vi "acquire_dataMultiAxis.vi"(0 "Freq_i":dbl format="%#_13g", 5 "FPGA VI Reference in":refnum<k20>, 7 "error in":errorcluster, 9 "Nsamps_i":i32, 11 "data (sin wave) in":dbl[](array[numeric])) -> (2 "Elements Remaining":i32=1, 4 "FPGA VI Reference Out":refnum<k20>, 6 "error IO":errorcluster, 10 "output cluster":cluster{"z-err data":dbl[], "u_z-data":dbl[]}, 15 "elements left":i32=1)   [LabVIEW 2017]
uses:
  <vilib>/Utility/error.llb/Error Cluster From Error Code.vi
  <vilib>/rvi/errors/niLvFpgaAdjustHostInterfaceError.vi
  <vilib>/rvi/interface/nirviMethod/nirviMethod.xnode
  <vilib>/rvi/errors/niLvFpgaMergeErrorWithErrorCode.vi
  <vilib>/FPGAPlugInAG/Dynamic/niLvFpga_ReadFifo_Dynamic.vi
  <vilib>/FPGAPlugInAG/Dynamic/niLvFpga_WriteFifo_Dynamic.vi
panel:
  out "x+y 2":i32
  out "appended array":i32[](array[numeric])
  out "Numeric 3":i32
  out "Numeric 2":i32
  out "x+y":i32
  out "Numeric":i32
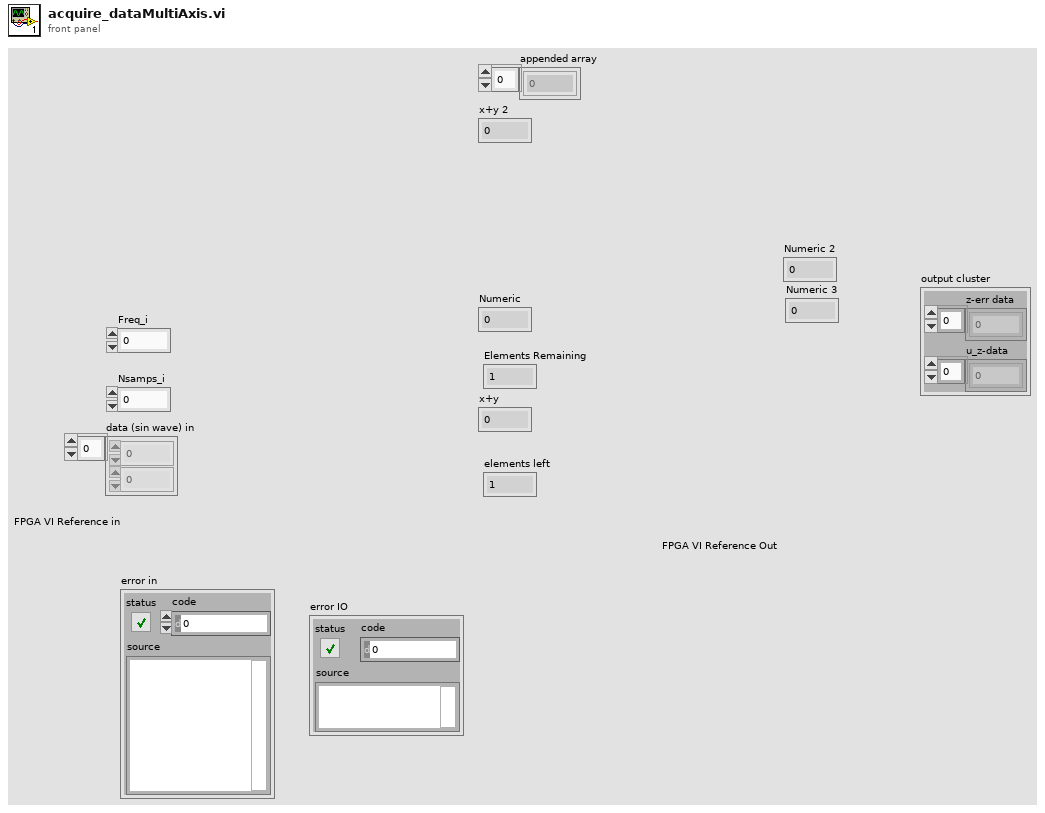
[diagram p1: front panel]
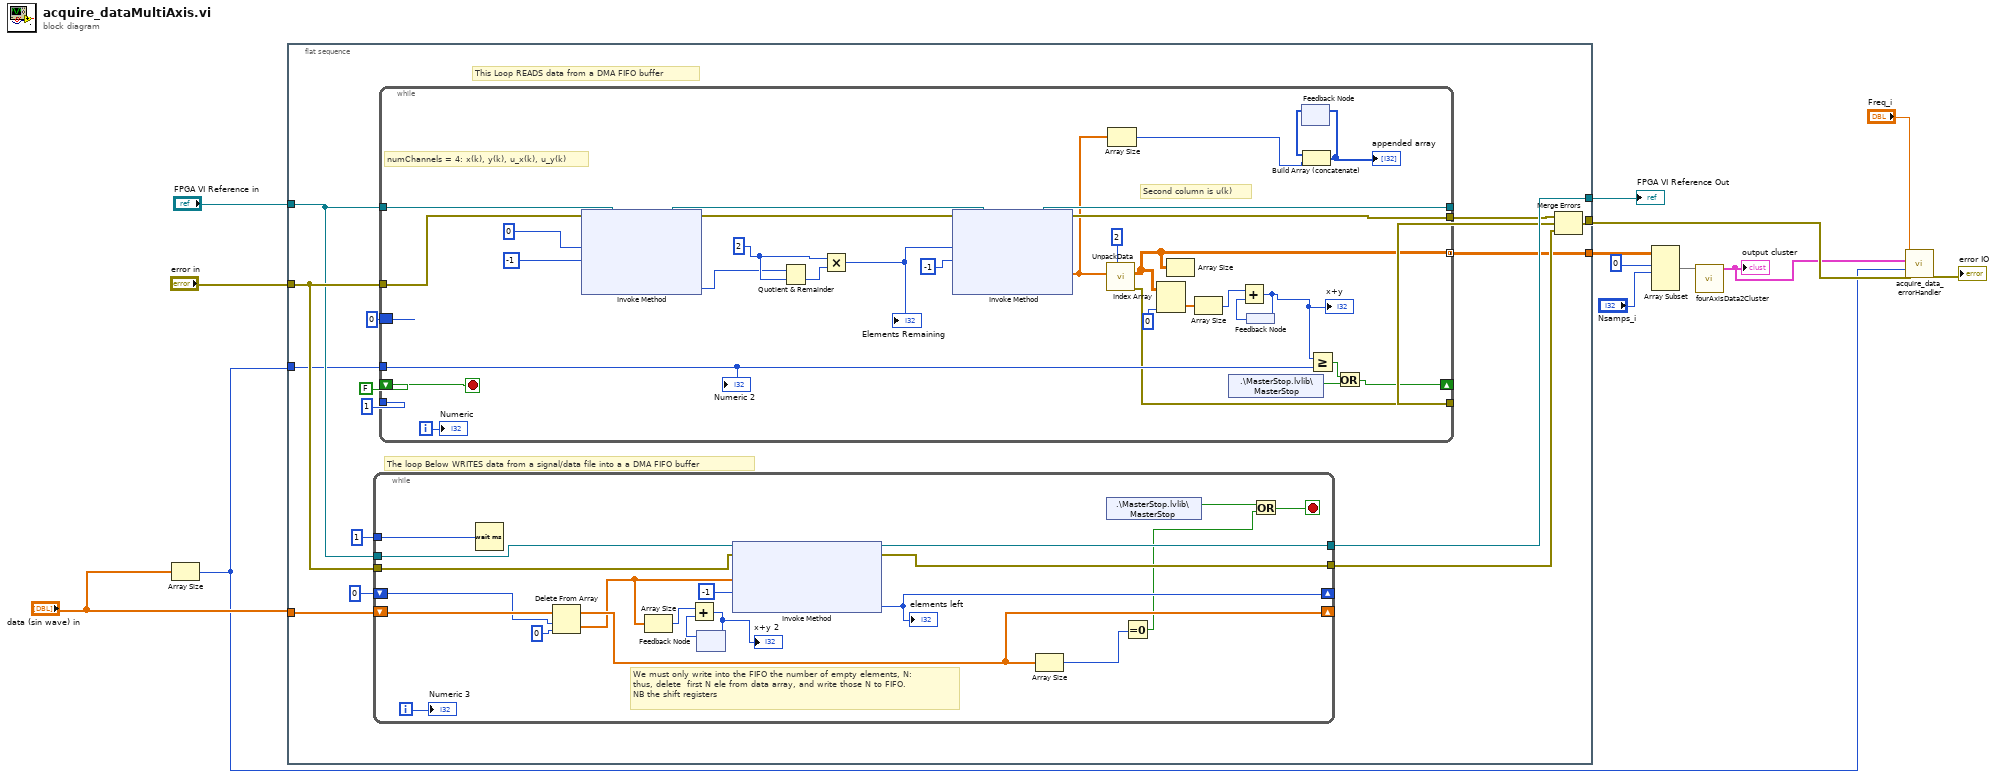
[diagram p0: block diagram]
diagram:
  n1 = Array Size(array="data (sin wave) in") -> (size(s)=w2:i32)
  n2 = flat-sequence {
    tunnel: "data (sin wave) in" -> [w20]
    tunnel: "error in" -> [w22]
    tunnel: "FPGA VI Reference in" -> [w21]
    tunnel: [w28] -> w3
    tunnel: [w27] -> w11
    tunnel: w2 -> [w18]
    tunnel: [w14] -> w9
    frame #0 {
      # "This Loop READS data from a DMA FIFO buffer"
      # "The loop Below WRITES data from a signal/data file into a a DMA FIFO buffer"
      n3 = while {
        tunnel: [w76] -> w28
        tunnel: [w77] -> w17
        tunnel: 1 -> [w79]
        shift-right: [w70] -> _
        shift-left: u32 0 ("Empty Elements Remaining") -> [w75]
        shift-right: [w74] -> _
        shift-left: w20 -> [w78]
        tunnel: w21 -> [w73]
        tunnel: w22 -> [w72]
        i -> [w71]
        stop <- w64 stop-if-true
        # "We must only write into the FIFO the number of empty elements, N:\nthus, delete  first N ele from data array, and write those N to FIFO.\nNB the shift registers"
        n4 = Wait (ms)(milliseconds to wait=w79) -> ()  [unwired: 1 out]
        n5 = Delete From Array(array=w78, length=w75, index=0) -> (deleted portion=w61:dbl[], array with subset deleted=w74:dbl[])
        n6 = Array Size(array=w61) -> (size(s)=w62:i32)
        n7 = feedback #1() -> (w63:i32)  [unwired: 1 in]
        n8 = Add(x=w62, y=w63) -> (x+y=w60:i32)
        "x+y 2" <- w60
        n9 = feedback-in #1(w60) -> ()
        n10 = xnode "Invoke Method"("FPGA VI Reference In"=w73, "error in"=w72, "Data"=w61, "Timeout (ms)"=-1) -> ("FPGA VI Reference Out"=w76:refnum<k20>, "error out"=w77:errorcluster, "Empty Elements Remaining"=w70:u32)
        "elements left" <- w70
        n11 = Array Size(array=w74) -> (size(s)=w67:i32)
        n12 = shared-variable ".\\MasterStop.lvlib\\MasterStop"() -> (w66:bool)  [unwired: 1 in, 1 out]
        n13 = Equal To 0?(x=w67) -> (x = 0?=w65:bool)
        n14 = Or(x=w66, y=w65) -> (x .or. y?=w64:bool)
        "Numeric 3" <- w71
      }
      n15 = while {
        tunnel: [w57] -> w26
        tunnel: [w58] -> _
        tunnel: u32 1 -> [_]
        tunnel: w18 -> [w56]
        shift-right: [w38] -> _
        shift-left: FALSE -> [w55]
        tunnel: w21 -> [w50]
        tunnel: w22 -> [w49]
        tunnel: [w41] -> w16
        border: u32 0 -> [_]
        tunnel: [w33] -> w14 mode=concatenating
        i -> [w48]
        stop <- w55 stop-if-true
        w45 = 2
        # "numChannels = 4: x(k), y(k), u_x(k), u_y(k)"
        # "Second column is u(k)"
        n16 = xnode "Invoke Method"("FPGA VI Reference In"=w50, "error in"=w49, "Number of Elements"=u32 0 ("Timeout (ms)"), "Timeout (ms)"=-1) -> ("FPGA VI Reference Out"=w52:refnum<k20>, "error out"=w59:errorcluster, "Elements Remaining"=w44:u32)  [unwired: 1 out]
        n17 = Quotient & Remainder(x=w44, y=w45) -> (floor(x/y)=w46:u32)  [unwired: 1 out]
        n18 = Multiply(x=w45, y=w46) -> (x*y=w35:u32)
        "Elements Remaining" <- w35
        n19 = xnode "Invoke Method"("FPGA VI Reference In"=w52, "error in"=w59, "Number of Elements"=w35, "Timeout (ms)"=-1) -> ("FPGA VI Reference Out"=w58:refnum<k20>, "error out"=w57:errorcluster, "Data"=w30:sgl[])  [unwired: 1 out]
        n20 = call "UnpackData.vi"("NumChannels"=2, "1D Data In"=w30) -> ("error Out"=w41:errorcluster, "2D Data Out"=w33:dbl[][])  [unwired: 8 in]
        n21 = Array Size(array=w30) -> (size(s)=w29:i32)
        n22 = Index Array(array=w33, index (col)=0) -> (element=w34:dbl[])  [unwired: 1 in]
        n23 = Array Size(array=w33) -> ()  [unwired: 1 out]
        n24 = Array Size(array=w34) -> (size(s)=w39:i32)
        n25 = shared-variable ".\\MasterStop.lvlib\\MasterStop"() -> (w36:bool)  [unwired: 1 in, 1 out]
        n26 = feedback #2() -> (w42:u32)
        n27 = Add(x=w39, y=w42) -> (x+y=w43:u32)
        "x+y" <- w43
        n28 = feedback-in #2(w43) -> ()
        n29 = feedback #3() -> (w32:i32[])  [unwired: 1 in]
        n30 = Build Array (concatenate)(w32, w29) -> (w31:i32[])
        "appended array" <- w31
        n31 = feedback-in #3(w31) -> ()
        n32 = Greater Or Equal?(x=w43, y=w56) -> (x >= y?=w37:bool)
        n33 = Or(x=w37, y=w36) -> (x .or. y?=w38:bool)
        "Numeric" <- w48
        "Numeric 2" <- w56
      }
      n34 = Merge Errors(w26, w16, w17) -> (w27:errorcluster)
    }
  }
  n35 = Array Subset(array=w9, index (row)=0 ("index"), length (row)="Nsamps_i") -> (w6:dbl[][])  [unwired: 2 in]
  n36 = call "fourAxisData2Cluster.vi"("2D Data Out in"=w6) -> ("output cluster"=w1:cluster{"z-err data":dbl[], "u_z-data":dbl[]})  [unwired: 10 in]
  "output cluster" <- w1
  n37 = call "acquire_data_errorHandler.vi"("error in (no error)"=w11, "length Sin wave Input"=w2, "input cluster"=w1, "Freq_i"="Freq_i") -> ("error out"=→"error IO":errorcluster)  [unwired: 7 in]
  "FPGA VI Reference Out" <- w3
